vi "Config.vi"() -> (3 "Show Console":bool=TRUE)   [LabVIEW 2013, in "Advanced Plotting Toolkit.lvlib"]
doc: "Basic configuration parameters for the Toolkit. To change settings, alter the control values and then right-click and use \"Data Operations->Make Current Values Default\"."
uses:
  Advanced Plotting Toolkit.lvlib
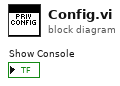
[diagram p0: block diagram]
diagram:
